vi "DataSender.vi"() -> ()   [LabVIEW 2015]
uses:
  <vilib>/userdefined/High Color/IMAQdx.ctl
  <vilib>/DAQmx/read.llb/DAQmx Read (Analog 2D DBL NChan NSamp).vi
  <vilib>/DAQmx/configure/timing.llb/DAQmx Timing (Sample Clock).vi
  <vilib>/DAQmx/miscellaneous.llb/DAQmx Fill In Error Info.vi
  <vilib>/vision/driver/NI_Vision_Acquisition_Software.lvlib
panel:
  in  "Tab Control 2":T1(tab)
  out "Video Data Acquisition Loop":T2(plugin-control)
  out "Video Display Loop":T2(plugin-control)
  out "Video Save Loop":T2(plugin-control)
  out "AI DAQ Loop":dbl[][](graph)
  out "AI UDP Send & AI Save Loop":dbl[][](graph)
  out ".tdms-file path":path
  out ".bin-file path":path
  out ".avi-file path":path
  in  "Save Binary file":bool
  in  "Save AVI file":bool
  in  "Record Button":bool
  in  "Recording number":dbl
  in  "File path":path
  in  "Stop Button":bool
  in  "Camera module":T3
  # "File paths"
  # "1. Select camera module\n2. Select file path and recording number\n3. Select what file-types to save\n4. Start program\n5. Select \"Record\""
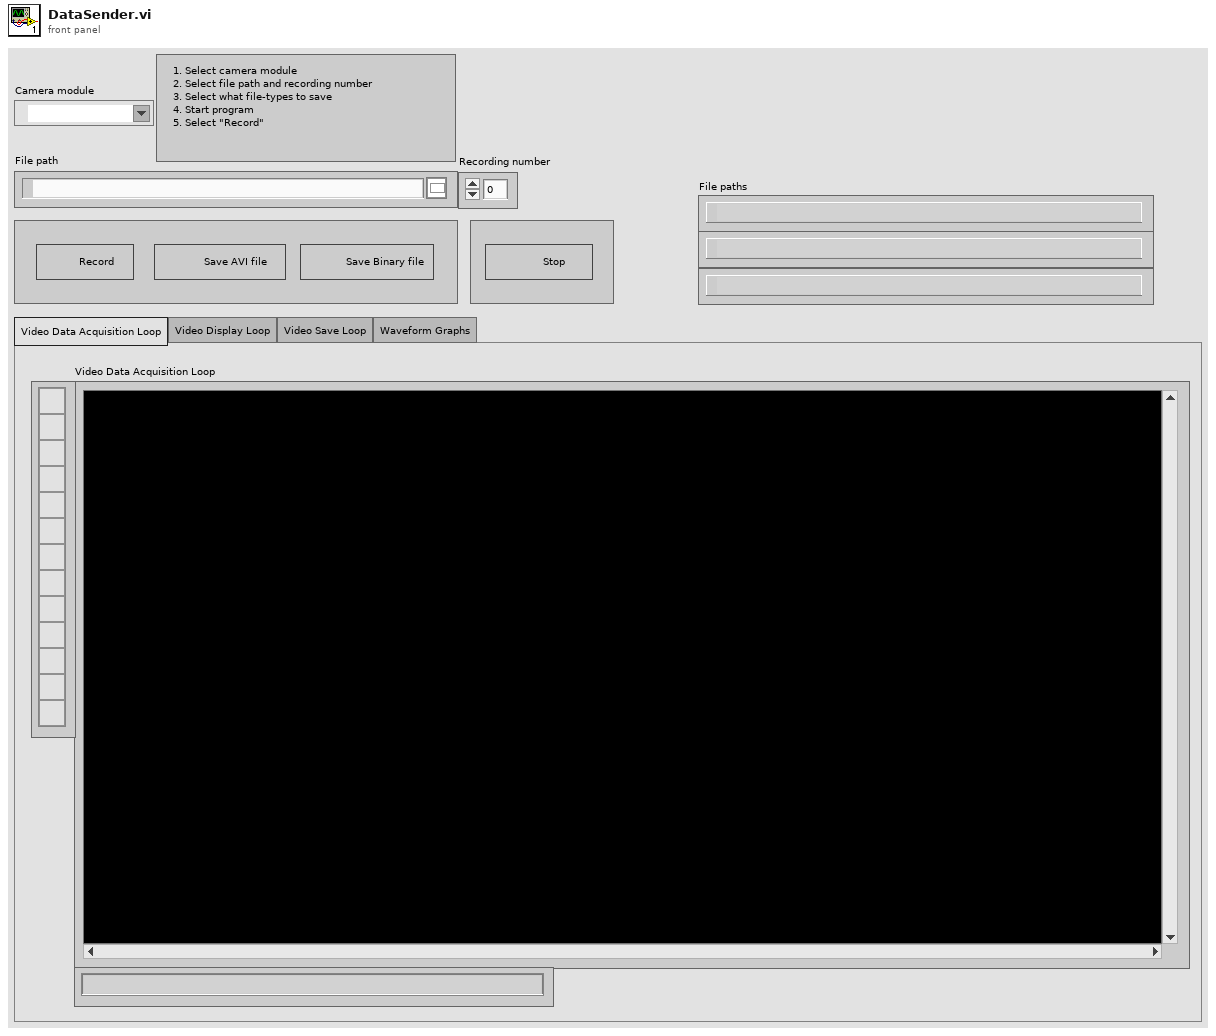
[diagram p1: front panel]
types:
  T1 = enum32{"Video Data Acquisition Loop", "Video Display Loop", "Video Save Loop", "Waveform Graphs"}
  T2 = typedef "IMAQ Image.ctl" = refnum<image>
  T3 = typedef "IMAQdx.ctl" = refnum<k21>
  T4 = enum16{"open", "open or create", "create or replace", "create", "open (read-only)"}
  T5 = enum16{"open", "replace", "create", "open or create", "replace or create", "replace or create with confirmation"}
  T6 = typedef "Image Type" = u32
  T7 = typedef "IMAQ AVI2 Refnum.ctl" = refnum<k20>
  T8 = enum16{"big-endian, network order", "native, host order", "little-endian"}
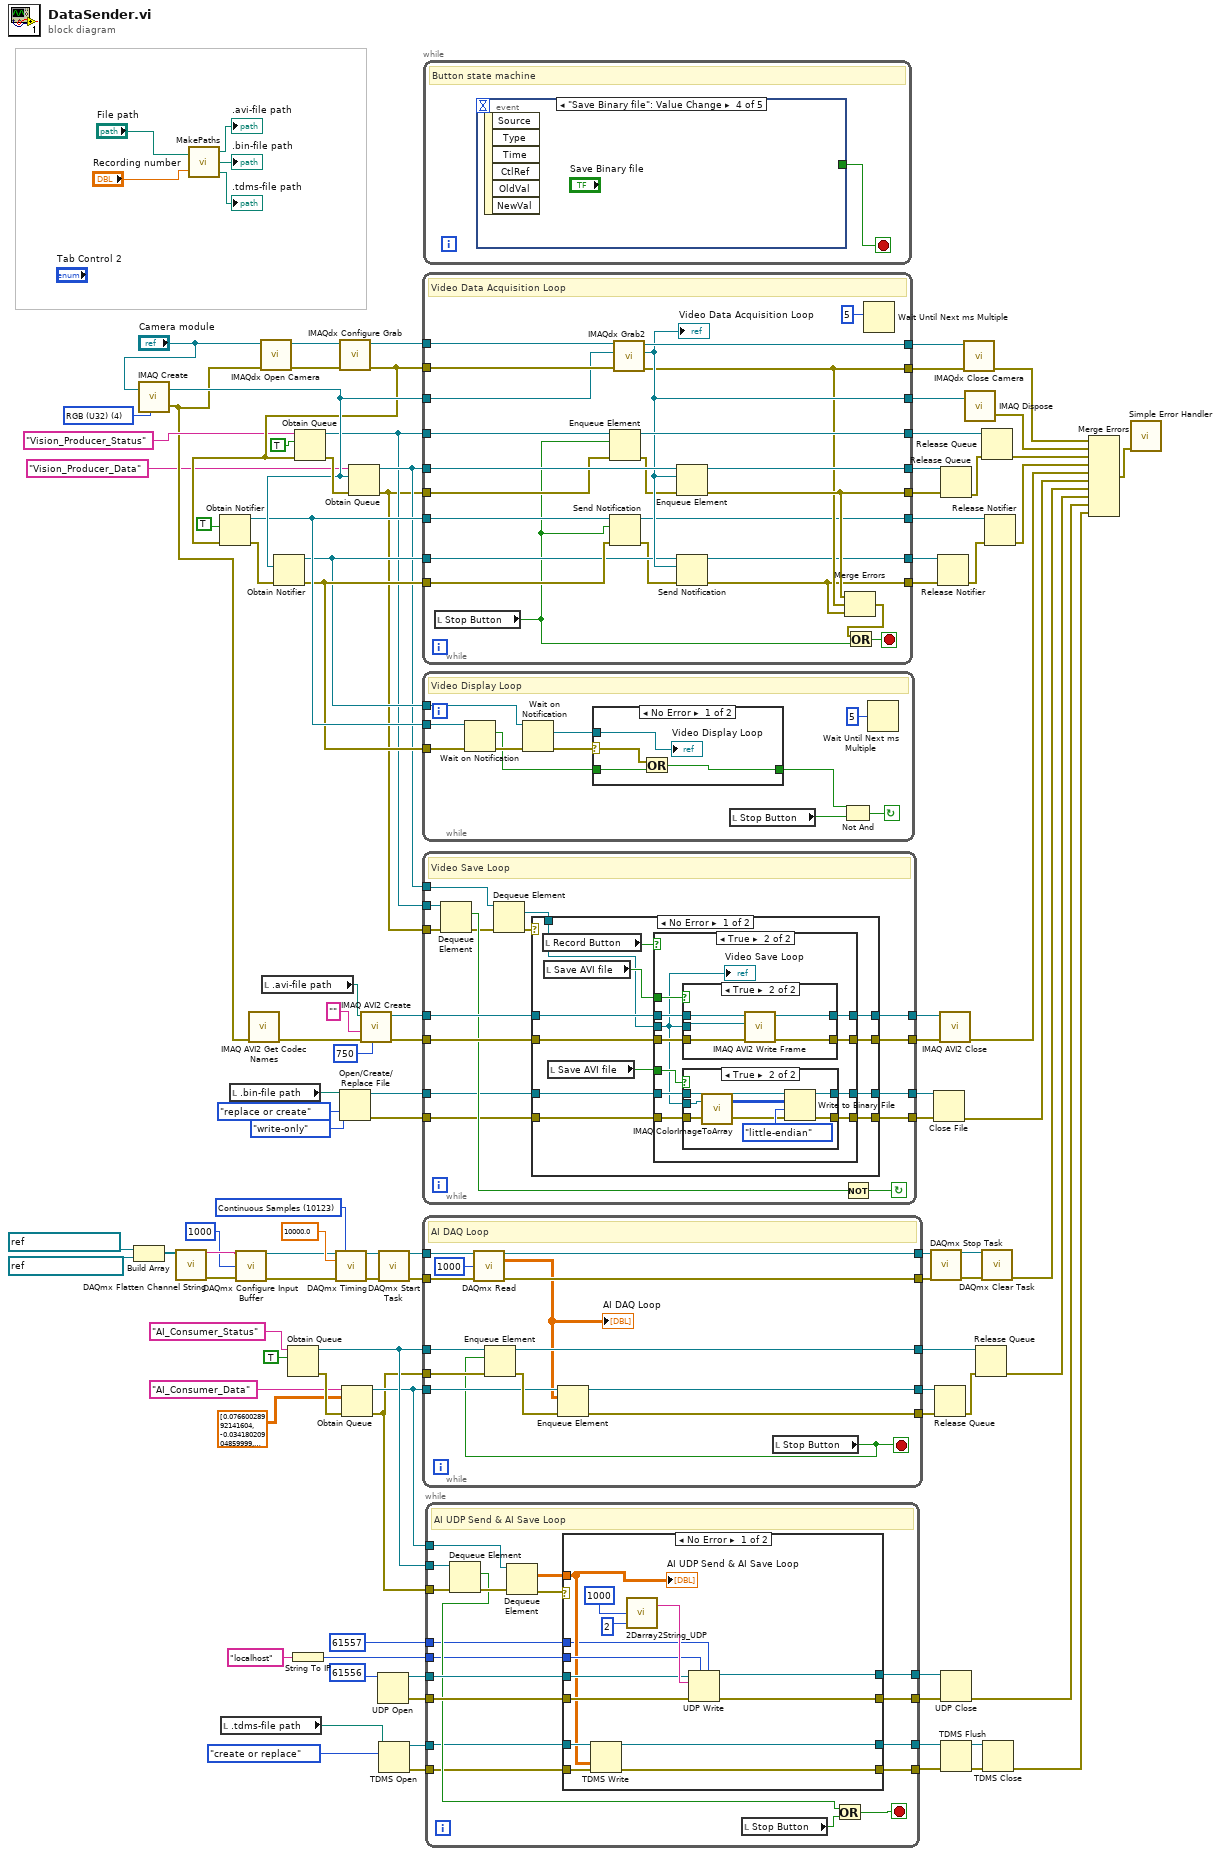
[diagram p0: block diagram]
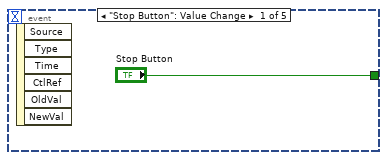
[diagram p2: hidden frame]
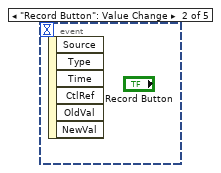
[diagram p3: hidden frame]
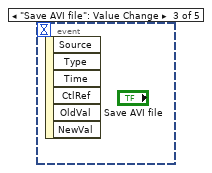
[diagram p4: hidden frame]
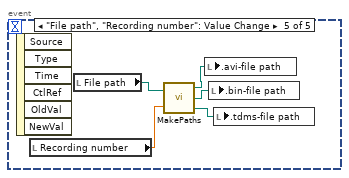
[diagram p5: hidden frame]
diagram:
  w52 = 10123 items=["Finite Samples"=10178, "Continuous Samples"=10123, "Hardware Timed Single Point"=12522] ("sample mode")
  w107 = T6 4 items=["Grayscale (U8)", "Grayscale (I16)", "Grayscale (SGL)", "Complex (CSG)", "RGB (U32)", "HSL (U32)", "RGB (U64)", "Grayscale (U16)"] ("Image Type")
  n1 = Build Array(refnum<k21> "DAQmx_USB_a0" ("global virtual channels"), refnum<k21> "DAQmx_USB_ai1" ("global virtual channels")) -> (w22:refnum<k21>[])
  n2 = call "IMAQ Create"("Image Name"="Camera module", "Image Type"=w107) -> ("New Image"=w85:T2, "error out"=w37:errorcluster)  [unwired: 3 in]
  n3 = call <vilib>:"DAQmx Flatten Channel String.vi"("names in"=w22) -> ("names out"=w21:string, "error out"=w23:errorcluster)  [unwired: 13 in]
  n4 = call "MakePaths.vi"("File path"="File path", "File name index"="Recording number") -> (".avi-file path"=→".avi-file path":path, ".bin-file path"=→".bin-file path":path, ".tdms-file path"=→".tdms-file path":path)
  n5 = local read ".tdms-file path"() -> (w11:path)
  n6 = local read ".bin-file path"() -> (w62:path)
  n7 = call <vilib>:"DAQmx Configure Input Buffer.vi"("task/channels in"=w21, "buffer size (in samples per channel)"=u32 1000, "error in"=w23) -> ("task out"=w25:refnum<k21>, "error out"=w26:errorcluster)  [unwired: 11 in]
  n8 = call "IMAQ AVI2 Get Codec Names"("error in (no error)"=w37) -> ("error out"=w71:errorcluster)  [unwired: 9 in, 1 out]
  n9 = call <vilib>:"IMAQdx Open Camera.vi"("error in"=w37, "Session In"="Camera module") -> ("error out"=w92:errorcluster, "Session Out"=w108:T3)  [unwired: 8 in]
  n10 = local read ".avi-file path"() -> (w68:path)
  n11 = Obtain Queue(name (unnamed)="AI_Consumer_Status", element data type=TRUE) -> (queue out=w29:refnum<queue>, error out=w45:errorcluster)  [unwired: 3 in, 1 out]
  n12 = String To IP(1:"localhost" ("name")) -> (0:w12:u32)
  n13 = call-poly <vilib>:"DAQmx Timing.vi"("task/channels in"=w25, "sample mode"=w52, "rate"=10000.0, "error in"=w26) -> ("task out"=w49:refnum<k21>, "error out"=w48:errorcluster)  [unwired: 10 in]
  n14 = call <vilib>:"IMAQdx Configure Grab.vi"("error in"=w92, "Session In"=w108) -> ("error out"=w76:errorcluster, "Session Out"=w106:T3)  [unwired: 8 in]
  n15 = Obtain Notifier(notification data type=TRUE, error in (no error)=w76) -> (notifier out=w83:refnum<notifier>, error out=w89:errorcluster)  [unwired: 2 in, 1 out]
  n16 = Obtain Notifier(notification data type=w85, error in (no error)=w89) -> (notifier out=w81:refnum<notifier>, error out=w82:errorcluster)  [unwired: 2 in, 1 out]
  n17 = Obtain Queue(name (unnamed)="Vision_Producer_Status", element data type=TRUE, error in (no error)=w76) -> (queue out=w78:refnum<queue>, error out=w101:errorcluster)  [unwired: 2 in, 1 out]
  n18 = Open/Create/Replace File(file path (use dialog)=w62, operation (0:open)=T5."replace or create", access (0:read/write)=enum16{"read/write", "read-only", "write-only"}."write-only") -> (refnum out=w59:refnum<file>, error out=w58:errorcluster)  [unwired: 3 in, 1 out]
  n19 = Obtain Queue(name (unnamed)="AI_Consumer_Data", element data type=dbl[][] [[0.07660028992141604, -0.03418020904859999, 0.11871519035629816, 0.020752269779507133, 0.03143358510719463, 0.10772869459067674, 0.0997940032043946, 0.28046082246128023, 0.10498207064927138, 0.38056000610360874, 0.18097199969481956, 0.30823224231326773, 0.311284046692607, 0.3820859082932784, 0.3564507515068284, 0.4528877698939498, 0.5416952773327229, 0.47669184405279624, 0.6939803158617532, 0.6073090714885175, 0.5560387579156176, 0.5215533684290837, 0.6710917830167086, 0.8279545281147478, 0.7623407339589532, 0.8804455634393835, 0.7989623865110247, 0.942397192339971, 0.7824826428625925, 0.9246967269398032, 0.831616693369955, 0.9442282749675746, 0.9085221637293049, 1.0220492866407263, 1.164568551155871, 0.9750514991989013, 1.0428015564202335, 1.1123826962691692, 1.1206225680933852, 1.1956969558251316, 1.3278400854505226, 1.2719920653086136, 1.3226520180056458, 1.2417792019531548, 1.4630350194552528, 1.2643625543602655, 1.453879606317235, 1.3699549858854048, 1.4087129015030138, 1.4785992217898833, 1.5063706416418707, 1.3907072556649118, 1.6791027695124743, 1.6565194171053637, 1.7166399633783473, 1.58632791638056, 1.7196917677576868, 1.6055542839703976, 1.7880521858548868, 1.7206073090714886, 1.7761501487754634, 1.799649042496376, 1.8023956664377814, 1.731898985275044, 1.9461356527046616, 2.069428549629969, 1.816433966582742, 2.017242694743267, 2.0242618448157472, 1.9760433356221867, 1.9491874570840009, 2.1002517738612956, 2.128023193713283, 2.277256427862974, 2.053864347295338, 2.1911955443656064, 2.317235065232319, 2.3770504310673686, 2.178377965972381, 2.2287327382314794, 2.396887159533074, 2.464637216754406, 2.3141832608529795, 2.3154039826047152, 2.5094987411306935, 2.540627145799954, 2.630655374990463, 2.4350347142748148, 2.4145876249332416, 2.5314717326619363, 2.699931334401465, 2.6623941405355915, 2.75394827191577, 2.589456015869383, 2.705119401846342, 2.656290531776913, 2.6089875638971542, 2.681620508125429, 2.7405203326466774, 2.8427557793545435, 2.938887617303731, 2.9669642175936524, 2.895551995117113, 2.7850766765850308, 3.0130464637216754, 2.8589303425650416, 2.928816662851911, 3.040817883573663, 3.0261692225528343, 2.976729991607538, 3.0283054856183718, 3.0075532158388647, 3.002059967956054, 3.0850690470740827, 3.2593270771343557, 3.1540398260471503, 3.087815671015488, 3.2187380788891433, 3.2001220721751737, 3.241626611734188, 3.4302281223773554, 3.1973754482337684, 3.265430685893034, 3.4296177615014876, 3.3450827801937897, 3.526970321202411, 3.5153734645609216, 3.4726482032501718, 3.36919203479057, 3.4863813229571985, 3.556267643244068, 3.6014343480582895, 3.603875791561761, 3.6066224155031663, 3.5236133363851376, 3.493400473029679, 3.744258793011368, 3.5324635690852215, 3.7558556496528572, 3.8290989547570002, 3.594720378423743, 3.6734569314106964, 3.756466010528725, 3.838864728770886, 3.774166475928893, 3.744258793011368, 3.7390707255664912, 3.833981841763943, 3.9075303273060196, 3.88891432059205, 3.966124971389334, 4.026245517662318, 4.005798428320745, 3.8962386511024643, 3.969787136644541, 4.137026016632334, 3.931334401464866, 4.099183642328526, 4.063172350652323, 4.090638590066376, 3.953612573434043, 4.0650034332799265, 4.038147554741741, 3.9975585564965286, 4.2905317769131, 4.171206225680934, 4.151674677653163, 4.323491264209964, 4.237125200274662, 4.368352788586251, 4.19806210421912, 4.1486228732738235, 4.183108262760357, 4.332341496910048, 4.269779507133593, 4.409857328145266, 4.216983291371023, 4.40161745632105, 4.5053788052185855, 4.436102845807584, 4.417486839093614, 4.305790798809796, 4.425116350041963, 4.365606164644846, 4.4336614023041125, 4.476081483176928, 4.554512855725948, 4.455634393835355, 4.4507515068284125, 4.549324788281071, 4.633249408712902, 4.575570305943389, 4.545052262149996, 4.455329213397421, 4.415960936903945, 4.490424963759823, 4.525520714122225, 4.4925612268253605, 4.654612039368277, 4.630197604333563, 4.563057907988098, 4.6936751354238195, 4.674448767833982, 4.648203250171664, 4.507515068284123, 4.674143587396048, 4.6323338673991, 4.5642786297398334, 4.591744869153887, 4.573434042877851, 4.666208896009766, 4.598764019226367, 4.823376821545739, 4.679026474402991, 4.830090791180285, 4.592355230029755, 4.864576180666819, 4.64240482185092, 4.616464484626535, 4.812390325780117, 4.698252841992828, 4.677500572213321, 4.768139162279698, 4.8490119783321886, 4.8825818265049215, 4.85145342183566, 4.77607385366598, 4.796520943007553, 4.892957961394675, 4.85999847409781, 4.763561455710689, 4.82429236285954, 4.950942244602121, 4.891432059205005, 4.860608834973678, 4.933241779201953, 4.741283283741512, 4.877393759060045, 4.764476997024491, 4.901503013656825, 4.71625848783093, 4.831921873807889, 4.986953536278325, 4.716868848706798, 4.887769893949798, 4.776989394979782, 4.990310521095598, 4.89570458533608, 4.705882352941177, 4.856946669718471, 4.81025406271458, 4.891737239642939, 4.925917448691539, 4.739757381551843, 4.767223620965896, 4.990005340657664, 4.863050278477149, 4.704661631189441, 4.762645914396887, 4.789806973373007, 4.934157320515755, 4.819409475852598, 4.966811627374685, 4.874036774242771, 4.8865491721980625, 4.903028915846495, 4.89021133745327, 4.767223620965896, 4.914930952925918, 4.677805752651255, 4.7440299076829175, 4.680552376592661, 4.866407263294422, 4.70771343556878, 4.889906157015336, 4.743114366369116, 4.831006332494087, 4.8239871824216065, 4.873121232928969, 4.723582818341344, 4.722056916151675, 4.840161745632105, 4.747997253376059, 4.836194399938964, 4.643015182726788, 4.85145342183566, 4.7864499885557334, 4.635996032654307, 4.841077286945906, 4.824902723735408, 4.777294575417716, 4.802014190890364, 4.648508430609598, 4.67505912870985, 4.711070420386053, 4.606393530174715, 4.614023041123064, 4.52674143587396, 4.753795681696803, 4.671702143892577, 4.617380025940337, 4.568551155870908, 4.506904707408255, 4.516975661860075, 4.574959945067521, 4.4885938811322195, 4.5557335774776835, 4.4885938811322195, 4.430914778362707, 4.603341725795376, 4.604562447547112, 4.581368734264133, 4.336308842603189, 4.468757152666514, 4.499885557335775, 4.345464255741207, 4.417486839093614, 4.384222171358816, 4.541390096894789, 4.481574731059739, 4.428473334859236, 4.378423743038072, 4.479438467994202, 4.422674906538491, 4.192874036774243, 4.288090333409628, 4.200503547722591, 4.305180437933928, 4.235294117647059, 4.319218738078889, 4.301213092240787, 4.125429159990845, 4.195315480277714, 4.300907911802853, 4.147402151522088, 4.284733348592355, 4.133363851377127, 4.021057450217441, 4.023498893720912, 4.221560997940032, 4.223086900129702, 4.055237659266041, 4.167849240863661, 3.9319447623407338, 4.028992141603723, 4.078736552986953, 3.9942015716792554, 3.8776226443884947, 4.074158846417944, 4.0683604180972, 3.9047837033646142, 3.8791485465781643, 3.9948119325551232, 3.8907454032196536, 3.986572060730907, 3.6990920881971467, 3.8815899900816357, 3.678644998855573, 3.7973601892118714, 3.812924391546502, 3.7085526817730985, 3.7949187457084, 3.838559548332952, 3.6649118791485464, 3.551384756237125, 3.7839322499427785, 3.616388189517052, 3.714656290531777, 3.689631494621195, 3.60845349813077, 3.489127946898604, 3.467460135805295, 3.4009308003356984, 3.578545815213245, 3.403067063401236, 3.296253910124361, 3.5373464560921644, 3.262989242389563, 3.3157854581521327, 3.4476234073395897, 3.295338368810559, 3.291676203555352, 3.2065308613717862, 3.2382696269169147, 3.167467765316243, 3.143358510719463, 3.2733653772793163, 3.135118638895247, 3.2858777752346073, 3.023117418173495, 3.1204699778744183, 3.1274891279468986, 3.150682841229877, 2.92484931715877, 2.929732204165713, 3.083237964446479, 3.0472266727702753, 2.783245593957427, 3.0218966964217593, 2.994430457007706, 2.9498741130693524, 2.8110170138094146, 2.704509040970474, 2.808575570305943, 2.8140688181887543, 2.827801937895781, 2.6074616617074846, 2.750286106660563, 2.7563897154192416, 2.6706340123598076, 2.7063401235980775, 2.626688029297322, 2.520180056458381, 2.4972915236133364, 2.631876096742199, 2.52475776302739, 2.3300526436255438, 2.374914168001831, 2.469825284199283, 2.491187914854658, 2.434424353398947, 2.354467078660258, 2.2446021210040437, 2.404211490043488, 2.23422598611429, 2.136263065537499, 2.193636987869078, 2.030060273136492, 1.999542229343099, 2.120393682764935, 2.0276188296330204, 2.1680018310826275, 2.0743114366369118, 1.944914930952926, 1.8780804150453956, 1.7834744792858779, 1.9684138246738383, 1.9128709849698635, 1.9336232547493706, 1.9269092851148242, 1.735866330968185, 1.906157015335317, 1.6623178454261083, 1.7419699397268635, 1.7428854810406653, 1.684901197833219, 1.6226443884946975, 1.560387579156176, 1.4209201190203709, 1.3785000381475547, 1.5616083009079118, 1.3830777447165636, 1.509727626459144, 1.5597772182803082, 1.3995574883649957, 1.3528648813611048, 1.385824368657969, 1.4108491645685513, 1.2048523689631494, 1.2091248950942244, 1.0797283894102387, 1.2713817044327458, 1.0522621499961853, 1.134050507362478, 1.0794232089723048, 1.1801327534905013, 1.0730144197756923, 0.9848172732127871, 0.8236820019836728, 0.7989623865110247, 0.788891432059205, 0.9137102311741817, 0.9799343862058442, 0.7284657053482871, 0.7354848554207676, 0.6747539482719158, 0.8114747844663157, 0.7071030746929122, 0.6744487678339819, 0.6198214694438087, 0.5325398641947051, 0.7013046463721675, 0.6884870679789425, 0.48035400930800337, 0.5484092469672694, 0.3811703669794766, 0.36957351033798735, 0.43732356755931945, 0.2865644312199588, 0.28412298771648736, 0.29114213778896775, 0.27862973983367667, 0.21240558480201419, 0.16601815823605706, 0.06805523765926604, 0.24414435034714274, 0.13366903181506065, 0.2404821850919356, 0.2050812542915999, -0.04180971999694819, 0.09308003356984818, -0.09643701838712139, -0.06713969634546425, -0.05035477225909819, -0.05462729839017319, -0.05035477225909819, -0.2697795071335927, -0.24170290684367132, -0.27252613107499807, -0.13031204699778745, -0.16510261692225528, -0.4687571526665141, -0.39032578011749447, -0.45685511558709085, -0.4574654764629587, -0.5957122148470283, -0.5606164644846265, -0.3884946974898909, -0.6094453345540551, -0.6271457999542229, -0.63080796520943, -0.6561379415579461, -0.6671244373235675, -0.652475776302739, -0.8255130846112764, -0.8139162279697871, -0.8014038300144961, -0.8984512092774853, -0.74189364461738, -0.9982452124818799, -0.9579613946746014, -0.9988555733577478, -0.8593881132219425, -1.1035324635690853, -0.9225604638742657, -1.1737239642938888, -1.1590753032730603, -0.9674219882505531, -1.0986495765621425, -1.1221484702830549, -1.0571450370031281, -1.2698558022430761, -1.2961013199053941, -1.4267185473411155, -1.2512397955291066, -1.244831006332494, -1.433127336537728, -1.4721904325932709, -1.4773785000381476, -1.603723201342794, -1.4508278019378957, -1.6742198825055314, -1.6827649347676814, -1.5716792553597314, -1.6403448538948653, -1.6235599298084993, -1.8063630121309224, -1.7364766918440528, -1.582055390249485, -1.6394293125810635, -1.676356145571069, -1.910734721904326, -1.8982223239490348, -1.7389181353475243, -1.9183642328526742, -1.803616388189517, -1.9162279697871367, -1.915312428473335, -1.975127794308385, -2.1097123674372473, -1.9461356527046616, -2.2317845426108187, -2.14023041123064, -2.1054398413061723, -2.0706492713817046, -2.1255817502098115, -2.1045242999923706, -2.1631189440756846, -2.246738384069581, -2.226901655603876, -2.312962539101244, -2.4713511863889526, -2.5189593347066452, -2.38803692683299, -2.4365606164644844, -2.4753185320820936, -2.448767833981842, -2.5256733043411916, -2.6544594491493094, -2.5214007782101167, -2.4512092774853134, -2.67704280155642, -2.6504921034561684, -2.622415503166247, -2.849774929427024, -2.866254673075456, -2.8213931486991686, -2.828717479209583, -2.738078889143206, -2.7856870374608986, -2.8964675364309147, -2.815899900816358, -2.8586251621271077, -2.787518120088502, -3.0722514686808577, -3.0826276035706113, -2.891889829861906, -2.8891432059205004, -3.1573968108644235, -2.9633020523384452, -3.057602807660029, -3.0908674753948273, -3.030746929121843, -3.2504768444342718, -3.130235751888304, -3.2059205004959184, -3.212329289692531, -3.23247119859617, -3.365224689097429, -3.403067063401236, -3.446402685587854, -3.240711070420386, -3.438467994201572, -3.361257343404288, -3.49736781872282, -3.4125276569771876, -3.598687724116884, -3.3380636301213094, -3.4579995422293432, -3.4647135118638897, -3.5315480277714197, -3.5489433127336536, -3.570000762951095, -3.4784466315709164, -3.736324101625086, -3.6606393530174715, -3.5568780041199357, -3.600213626306554, -3.7164873731593806, -3.595025558861677, -3.8702983138780804, -3.851377126726177, -3.880064087891966, -3.8480201419089037, -3.747920958266575, -3.753109025711452, -3.9554436560616466, -3.8190280003051806, -3.884031433585107, -3.8620584420538644, -3.917906462195773, -3.8529030289158466, -3.812924391546502, -4.1199359121080334, -4.128480964370184, -4.096742198825055, -3.9047837033646142, -4.113832303349355, -4.086671244373235, -4.065613794155794, -4.173342488746472, -4.050965133134966, -3.9948119325551232, -4.123292896925307, -4.097047379262989, -4.0442511635004195, -4.334477759975585, -4.075989929045548, -4.352178225375753, -4.111696040283817, -4.356450751506828, -4.275577935454337, -4.158083466849775, -4.287785152971694, -4.282597085526818, -4.437628747997254, -4.436102845807584, -4.246890974288548, -4.320134279392691, -4.373235675593194, -4.480354009308003, -4.539253833829251, -4.389105058365759, -4.529182879377432, -4.440070191500725, -4.341191729610132, -4.560616464484626, -4.54383154039826, -4.615548943312733, -4.415045395590143, -4.4101625085832, -4.616159304188601, -4.566720073243305, -4.483405813687343, -4.581368734264133, -4.583199816891737, -4.43427176317998, -4.615854123750667, -4.563363088426032, -4.615243762874799, -4.571908140688182, -4.627450980392157, -4.779736018921187, -4.518501564049744, -4.691538872358282, -4.789806973373007, -4.590218966964217, -4.655222400244145, -4.624093995574883, -4.556038757915617, -4.606393530174715, -4.571297779812314, -4.587472343022812, -4.695201037613489, -4.617990386816205, -4.740672922865644, -4.670481422140841, -4.742809185931182, -4.631113145647364, -4.819409475852598, -4.729381246662089, -4.761425192645151, -4.822461280231937, -4.713511863889525, -4.695811398489357, -4.814526588845655, -4.7022201876859695, -4.859082932784008, -4.696421759365225, -4.85297932402533, -4.791027695124742, -4.8157473105973905, -4.687571526665141, -4.713817044327459, -4.810864423590448, -4.969558251316091, -4.80018310826276, -4.831311512932021, -4.984817273212787, -4.7525749599450675, -4.897535667963684, -4.961623559929809, -4.753490501258869, -4.872205691615167, -4.847486076142519, -4.817883573662928, -4.900587472343023, -4.854200045777065, -4.903944457160296, -4.8200198367284655, -4.993362325474937, -4.896620126649882, -4.703746089875639, -4.855725947966735, -4.834058136873426, -4.838330663004501, -4.774242771038376, -4.9539940489814605, -4.82429236285954, -4.739757381551843, -4.854505226214999, -4.872510872053101, -4.942092011902037, -4.973525597009232, -4.728160524910353, -4.694895857175555, -4.7318226901655605, -4.931105516136416, -4.868848706797894, -4.943617914091707, -4.905470359349966, -4.840161745632105, -4.799267566948958, -4.7022201876859695, -4.857251850156405, -4.6939803158617535, -4.860914015411612, -4.653086137178607, -4.790722514686808, -4.794384679942016, -4.798046845197223, -4.82581826504921, -4.658274204623484, -4.607614251926451, -4.85297932402533, -4.8578622110322724, -4.712901503013657, -4.730296787975891, -4.574349584191653, -4.669565880827039, -4.673228046082246, -4.770885786221103, -4.737926298924239, -4.6494239719234, -4.799267566948958, -4.641794460975052, -4.579842832074464, -4.753185320820935, -4.682688639658198, -4.764171816586557, -4.542000457770657, -4.615548943312733, -4.549324788281071, -4.585641260395208, -4.630197604333563, -4.673838406958114, -4.5725185015640495, -4.510872053101396, -4.38605325398642, -4.4043640802624555, -4.599984740978103, -4.6436255436026554, -4.46845197222858, -4.57099259937438, -4.594796673533226, -4.542000457770657, -4.450141145952545, -4.486152437628748, -4.285954070344091, -4.285954070344091, -4.325932707713435, -4.486152437628748, -4.433051041428245, -4.457160296025025, -4.333867399099717, -4.315556572823682, -4.303349355306325, -4.432135500114443, -4.286869611657893, -4.327458609903105, -4.361943999389639, -4.086976424811169, -4.220340276188296, -4.09399557488365, -4.272220950637064, -4.114747844663157, -4.249027237354086, -4.130922407873656, -4.011596856641489, -4.056458381017777, -4.238345922026398, -4.133058670939193, -4.198367284657054, -4.042114900434882, -3.8873884184023804, -4.023804074158846, -4.130006866559854, -3.9472037842374306, -3.8245212481879913, -3.9163805600061035, -3.8367284657053484, -3.859616998550393, -3.8159761959258414, -3.8867780575265125, -3.8443579766536966, -3.7595178149080644, -3.786068513008316, -3.8614480811779965, -3.8525978484779126, -3.613031204699779, -3.7506675822079805, -3.615777828641184, -3.624322880903334, -3.5754940108339057, -3.5629816128786147, -3.7839322499427785, -3.6862745098039214, -3.71099412527657, -3.671625848783093, -3.6853589684901196, -3.4448767833981844, -3.5205615320057984, -3.59136339360647, -3.458304722667277, -3.312428473334859, -3.3868925001907377, -3.4857709620813306, -3.3112077515831233, -3.347829404135195, -3.42748149843595, -3.4644083314259557, -3.1815060654612037, -3.2062256809338523, -3.3627832455939575, -3.2895399404898145, -3.1119249256122683, -3.105516136415656, -3.096971084153506, -3.096971084153506, -3.134813458457313, -3.1024643320363166, -3.1100938429846647, -3.0304417486839093, -2.972457465476463, -3.0823224231326773, -2.862287327382315, -2.98619058518349, -3.0469214923323413, -2.860761425192645, -2.9132524605172807, -2.771343556878004, -2.9053177691309986, -2.6977950713359276, -2.6501869230182344, -2.6746013580529486, -2.75547417410544, -2.725871671625849, -2.631876096742199, -2.6507972838941023, -2.7148851758602275, -2.4884412909132525, -2.5433737697413594, -2.5137712672617685, -2.4713511863889526, -2.392004272526131, -2.563210498207065, -2.5473411154345005, -2.558022430762188, -2.2708476386663614, -2.444190127412833, -2.4243533989471273, -2.4386968795300223, -2.1640344853894864, -2.205233844510567, -2.341039139391165, -2.3074692912184327, -2.3044174868390934, -2.0364690623331043, -2.161287861448081, -1.999542229343099, -2.020904859998474, -2.0178530556191348, -1.876249332417792, -2.115205615320058, -2.0526436255436025, -1.9476615548943312, -1.8744182497901885, -1.9555962462806133, -1.8771648737315938, -1.8863202868696116, -1.8243686579690241, -1.7727931639581902, -1.6473640039673456, -1.6116578927290761, -1.7715724422064545, -1.530174715800717, -1.5463492790112154, -1.684596017395285, -1.5454337376974137, -1.5762569619287403, -1.5497062638284886, -1.3311970702677958, -1.4813458457312887, -1.3315022507057297, -1.3034256504158084, -1.2353704127565424, -1.4520485236896314, -1.3864347295338368, -1.313191424429694, -1.3415732051575493, -1.215228503852903, -1.2143129625391011, -1.2463569085221637, -1.1749446860456245, -1.1703669794766156, -1.1932555123216602, -1.0464637216754407, -0.8703746089875639, -0.8300907911802854, -0.8438239108873121, -0.959792477302205, -0.814526588845655, -0.7034409094377051, -0.7772945754177157, -0.7754634927901122, -0.8026245517662318, -0.6912336919203479, -0.5569542992294194, -0.6765850308995194, -0.5035477225909819, -0.6942854962996872, -0.5722133211261158, -0.4058899824521248, -0.6420996414129855, -0.4342717631799802, -0.42481116960402837, -0.341191729610132, -0.3909361409933623, -0.2868696116578927, -0.42786297398336764, -0.2859540703440909, -0.2743572137026017, -0.12756542305638208, -0.21637293049515527, -0.17120622568093385, -0.08819714656290532, -0.08941786831464103, -0.1718165865568017, 0.0311284046692607, 0.07171740291447318], [0.35065232318608375, 0.5310139620050355, 0.42481116960402837, 0.4852368963149462, 0.6454566262302587, 0.5859464408331426, 0.6515602349889372, 0.614023041123064, 0.5719081406881819, 0.8090333409628443, 0.5972381170366979, 0.7992675669489586, 0.7244983596551461, 0.9539940489814603, 0.7129015030136568, 0.8853284504463264, 0.7559319447623407, 1.0629434653238727, 1.1139085984588388, 1.0727092393377584, 0.899977111467155, 1.0861371786068512, 1.1740291447318227, 1.2591744869153887, 1.134050507362478, 1.142900740062562, 1.2561226825360494, 1.3156328679331655, 1.279011215381094, 1.2173647669184404, 1.1795223926146334, 1.4032196536202028, 1.4358739604791333, 1.4917219806210422, 1.4267185473411155, 1.4251926451514458, 1.560997940032044, 1.5188830395971618, 1.6870374608987564, 1.7169451438162813, 1.6778820477607386, 1.530174715800717, 1.5368886854352637, 1.6739147020675975, 1.8261997405966277, 1.6830701152056153, 1.7578393224994278, 1.718165865568017, 1.7502098115510796, 1.944914930952926, 1.7935454337376975, 1.9983215075913634, 1.8222323949034867, 2.013275349050126, 2.041962310215915, 2.032806897077897, 2.205233844510567, 2.1768520637827113, 1.9867246509498742, 2.1850919356069274, 2.0520332646677346, 2.1100175478751813, 2.2662699320973525, 2.1805142290379185, 2.3434805828946366, 2.408178835736629, 2.2781719691767757, 2.358434424353399, 2.461585412375067, 2.558327611200122, 2.3236438544289313, 2.5626001373311973, 2.502784771496147, 2.549477378500038, 2.4875257495994507, 2.5690089265278098, 2.626993209735256, 2.716716258487831, 2.7576104371709773, 2.5503929198138398, 2.7444876783398184, 2.7277027542534524, 2.8799877927824826, 2.6800946059357593, 2.8418402380407417, 2.7023727779049365, 2.8522163729304952, 2.771648737315938, 3.0417334248874646, 2.87357900358587, 2.8546578164339667, 2.8561837186236363, 3.105210955977722, 2.981307698176547, 2.9187457084000914, 3.19829098954757, 3.1665522240024413, 3.2089723048752576, 3.231860837720302, 3.1488517586022735, 3.3093766689555197, 3.3533226520180057, 3.282520790417334, 3.3344014648661022, 3.1778439002059966, 3.2346074616617075, 3.4396887159533076, 3.385976958876936, 3.426871137560082, 3.441519798580911, 3.2718394750896467, 3.303578240634775, 3.308155947203784, 3.4171053635461965, 3.5025558861676966, 3.658808270389868, 3.3969634546425573, 3.4787518120088503, 3.5040817883573663, 3.735713740749218, 3.551995117112993, 3.577630273899443, 3.6279850461585412, 3.608148317692836, 3.615777828641184, 3.595025558861677, 3.6737621118486303, 3.855344472419318, 3.8522926680399787, 3.6774242771038375, 3.794613565270466, 3.813839932860304, 3.9209582665751124, 4.005798428320745, 3.940489814602884, 3.768978408484016, 3.9890135042343786, 4.007324330510414, 3.9395742732890824, 3.881284809643702, 4.080872816052491, 3.999084458686198, 3.9157701991302356, 4.052796215762569, 4.065918974593728, 4.1739528496223395, 4.145571068894484, 4.128786144808118, 3.982299534599832, 4.221866178377966, 4.050659952697032, 4.138857099259938, 4.0988784618905925, 4.1879911497673, 4.22919050888838, 4.2746623941405355, 4.116273746852826, 4.169985503929198, 4.323796444647898, 4.30457007705806, 4.202029449912261, 4.351567864499885, 4.227664606698711, 4.226443884946975, 4.267338063630121, 4.473640039673457, 4.428168154421302, 4.3585870145723655, 4.476691844052796, 4.544441901274128, 4.586861982146944, 4.566720073243305, 4.599984740978103, 4.385137712672618, 4.558785381857023, 4.429388876173038, 4.5975432974746315, 4.414129854276341, 4.548104066529335, 4.641184100099184, 4.646677347981995, 4.667734798199436, 4.700999465934234, 4.552071412222476, 4.6018158236057065, 4.460517280842298, 4.736705577172503, 4.545967803463798, 4.695201037613489, 4.780956740672923, 4.516670481422141, 4.5557335774776835, 4.77454795147631, 4.725719081406882, 4.648813611047532, 4.715648126955062, 4.776379034103914, 4.570382238498512, 4.732433051041428, 4.852063782711528, 4.638437476157779, 4.679636835278859, 4.638742656595713, 4.6103608758678565, 4.850537880521858, 4.753490501258869, 4.627756160830091, 4.821545738918135, 4.639658197909514, 4.909742885481041, 4.906691081101702, 4.703440909437705, 4.696421759365225, 4.70771343556878, 4.921034561684596, 4.802014190890364, 4.836194399938964, 4.906080720225834, 4.7864499885557334, 4.86854352635996, 4.698252841992828, 4.758678568703746, 4.957656214236668, 4.775158312352178, 4.78461890592813, 4.75043869687953, 4.733043411917296, 4.867322804608224, 4.8325322346837565, 4.866407263294422, 4.698863202868696, 4.854810406652933, 4.9286640726329445, 4.703135728999771, 4.709544518196384, 4.838025482566567, 4.856641489280537, 4.813305867093919, 4.906691081101702, 4.8743419546807045, 4.985732814526589, 4.790722514686808, 4.9747463187609675, 4.880445563439384, 4.794995040817883, 4.69214923323415, 4.934157320515755, 4.873426413366903, 4.7348744945449, 4.694285496299687, 4.771496147096971, 4.946669718471046, 4.827954528114748, 4.792858777752346, 4.710154879072252, 4.686655985351339, 4.804455634393835, 4.834973678187228, 4.913099870298314, 4.725413900968948, 4.8783093003738465, 4.890516517891204, 4.928969253070878, 4.730296787975891, 4.75898374914168, 4.762951094834821, 4.671396963454643, 4.732127870603494, 4.799877927824826, 4.73334859235523, 4.837415121690699, 4.690318150606546, 4.787060349431601, 4.845349813076981, 4.664072632944229, 4.694895857175555, 4.563057907988098, 4.827954528114748, 4.821240558480201, 4.608529793240253, 4.689097428854811, 4.652475776302739, 4.642710002288854, 4.64240482185092, 4.744640268558785, 4.530098420691234, 4.49408712901503, 4.472114137483787, 4.664682993820096, 4.645761806668193, 4.579232471198596, 4.491340505073625, 4.61371786068513, 4.629587243457695, 4.3833066300450145, 4.4000915541313805, 4.599374380102235, 4.565804531929503, 4.55390249485008, 4.534065766384375, 4.419928282597086, 4.539253833829251, 4.319523918516823, 4.5297932402533, 4.553292133974212, 4.519111924925612, 4.343938353551537, 4.426642252231632, 4.380254825665675, 4.281071183337148, 4.221866178377966, 4.307011520561532, 4.347905699244678, 4.265812161440452, 4.208743419546807, 4.274967574578469, 4.267643244068055, 4.375371938658732, 4.288090333409628, 4.170901045243, 4.053711757076371, 4.307927061875334, 4.179140917067216, 4.22369726100557, 4.197146562905318, 4.227359426260777, 3.979247730220493, 3.9423208972304877, 4.1779201953154805, 3.975280384527352, 3.944762340733959, 4.042420080872816, 3.9145494773785, 4.114442664225223, 4.009460593575952, 3.9118028534370946, 4.051575494010834, 4.014953841458762, 3.940794995040818, 3.913939116502632, 3.8834210727092393, 3.8739604791332876, 3.8321507591363395, 3.8272678721293967, 3.817502098115511, 3.776913099870298, 3.735408560311284, 3.722590981918059, 3.6725413900968946, 3.6911573968108646, 3.6279850461585412, 3.680170901045243, 3.7174029144731824, 3.5025558861676966, 3.718623636224918, 3.539787899595636, 3.6435492484931715, 3.385671778439002, 3.591973754482338, 3.5938048371099414, 3.3792629892423895, 3.312428473334859, 3.488212405584802, 3.51293202105745, 3.3383688105592433, 3.2001220721751737, 3.2220950637064165, 3.4119172961013198, 3.2062256809338523, 3.39330128938735, 3.2382696269169147, 3.1525139238574806, 3.1662470435645074, 3.0869001297016863, 3.005416952773327, 3.1836423285267412, 3.061264972915236, 2.98466468299382, 3.0463111314564735, 3.019455252918288, 3.092698558022431, 2.895857175555047, 2.8061341268024718, 3.0536354619668877, 2.7579156176089112, 2.968490119783322, 2.7600518806744487, 2.8131532768749525, 2.8253604943923096, 2.861982146944381, 2.6535439078355076, 2.8479438467994203, 2.845502403295949, 2.754863813229572, 2.7862973983367665, 2.758525978484779, 2.601968413824674, 2.592813000686656, 2.6285191119249256, 2.561684596017395, 2.3974975204089417, 2.5705348287174794, 2.477759975585565, 2.293125810635538, 2.478675516899367, 2.4554818036163883, 2.452124818799115, 2.247348744945449, 2.1988250553139546, 2.145113298237583, 2.120393682764935, 2.0556954299229417, 2.2168307011520563, 2.264744029907683, 2.272068360418097, 2.20157167925536, 1.9339284351873045, 2.1002517738612956, 1.9214160372320135, 1.9729915312428474, 2.069733730067903, 2.0706492713817046, 1.9513237201495384, 1.952849622339208, 1.8731975280384527, 1.736171511406119, 1.8954757000076294, 1.7468528267338064, 1.7721828030823223, 1.7453269245441367, 1.5545891508354315, 1.6488899061570153, 1.5613031204699779, 1.6189822232394904, 1.454184786755169, 1.6427862973983367, 1.6260013733119707, 1.471274891279469, 1.5365835049973298, 1.3443198290989549, 1.5045395590142672, 1.369039444571603, 1.3925383382925154, 1.176775768673228, 1.1883726253147173, 1.3281452658884565, 1.1288624399176013, 1.1883726253147173, 1.258258945601587, 1.0473792629892424, 1.0754558632791638, 1.1029221026932174, 0.959487296864271, 0.8801403830014496, 0.9274433508812086, 1.0116731517509727, 0.8142214084077211, 0.7437247272449836, 0.7269398031586175, 0.9002822919050889, 0.7696650644693676, 0.8651865415426871, 0.6811627374685283, 0.814526588845655, 0.7879758907454032, 0.7650873579003585, 0.7174792095826658, 0.4620431830319677, 0.5673304341191729, 0.3799496452277409, 0.3781185626001373, 0.354009308003357, 0.5069047074082551, 0.3204394598306249, 0.24963759822995346, 0.281376363775082, 0.3054856183718624, 0.3689631494621195, 0.1330586709391928, 0.2316319523918517, 0.2975509269855802, 0.11169604028381781, 0.24811169604028382, 0.13977264057373923, 0.13031204699778745, -0.08789196612497138, 0.07690547035934997, -0.019836728465705347, -0.12695506218051422, -0.1815823605706874, -0.05493247882810712, -0.10620279240100709, -0.03143358510719463, -0.2887006942854963, -0.35919737544823377, -0.24719615472648204, -0.2801556420233463, -0.21332112611581597, -0.2307164110780499, -0.33600366216525523, -0.2859540703440909, -0.4217593652246891, -0.4528877698939498, -0.3915465018692302, -0.5136186770428015, -0.5838101777676051, -0.5676356145571069, -0.5795376516365301, -0.5828946364538033, -0.7769893949797818, -0.7058823529411765, -0.8987563897154193, -0.929579613946746, -0.8520637827115282, -0.9826810101472495, -0.8276493476768139, -0.8310063324940872, -0.9607080186160067, -0.8538948653391317, -1.0333409628442818, -0.8941786831464104, -1.1480888075074387, -1.1349660486762798, -1.1459525444419012, -1.0070954451819638, -1.2054627298390173, -1.1819638361181048, -1.091020065613794, -1.249713893339437, -1.3864347295338368, -1.437094682230869, -1.4874494544899672, -1.270771343556878, -1.2848096437018388, -1.4343480582894637, -1.6092164492256047, -1.4261081864652476, -1.376974135957885, -1.6690318150606547, -1.5042343785763332, -1.4767681391622798, -1.5243762874799724, -1.5286488136110474, -1.6821545738918136, -1.6549935149156938, -1.8393224994277866, -1.68886854352636, -1.8600747692072939, -1.8869306477454795, -2.0148012512397955, -1.9681086442359044, -2.0721751735713743, -1.8817425803006027, -2.1136797131303884, -2.1475547417410543, -1.9430838483253223, -2.08194094758526, -2.124361028458076, -2.153047989623865, -2.021820401312276, -2.1768520637827113, -2.0746166170748457, -2.1991302357518885, -2.379186694132906, -2.276035706111238, -2.4118410009918363, -2.2949568932631417, -2.367284657053483, -2.2497901884489204, -2.5424582284275576, -2.3147936217288474, -2.4426642252231634, -2.527504386968795, -2.6376745250629434, -2.6279087510490577, -2.6498817425803005, -2.461280231937133, -2.6968795300221258, -2.5943389028763257, -2.5702296482795455, -2.5516136415655755, -2.7780575265125504, -2.6205844205386435, -2.72983901731899, -2.7350270847638667, -2.8882276646066987, -2.8796826123445487, -2.973067826352331, -3.0337987335011825, -2.836652170595865, -2.890974288548104, -2.8973830777447165, -2.9706263828488595, -2.951400015259022, -3.1665522240024413, -3.1494621194781414, -3.0420386053253985, -3.257190814068818, -3.216601815823606, -3.0862897688258184, -3.1570916304264895, -3.2169069962615398, -3.117723353933013, -3.1964599069199666, -3.138170443274586, -3.2352178225375754, -3.2474250400549325, -3.2858777752346073, -3.483329518577859, -3.424429694056611, -3.3746852826733806, -3.3237201495384148, -3.3920805676356145, -3.5324635690852215, -3.5196459906919966, -3.653620202944991, -3.5526054779888607, -3.4351110093842983, -3.570611123826963, -3.6652170595864804, -3.493095292591745, -3.587701228351263, -3.7671473258564125, -3.72808422980087, -3.693598840314336, -3.6432440680552376, -3.6429388876173037, -3.790951400015259, -3.7625696192874036, -3.7296101319905395, -3.9337758449683373, -3.740291447318227, -3.8736552986953536, -3.8904402227817196, -3.945372701609827, -4.021972991531243, -4.067139696345464, -3.7894254978255892, -3.9862668802929733, -3.8275730525673306, -4.1113908598458835, -3.876096742198825, -4.1611352712291145, -4.040283817807278, -3.93011367971313, -4.113832303349355, -4.027771419851987, -4.14526588845655, -3.9884031433585108, -4.171511406118868, -4.015259021896696, -4.202029449912261, -4.144960708018616, -4.176699473563745, -4.107728694590676, -4.3793392843518735, -4.263065537499046, -4.231631952391852, -4.286259250782025, -4.151064316777295, -4.187075608453498, -4.192263675898375, -4.336919203479057, -4.458686198214695, -4.281071183337148, -4.3082322423132675, -4.519417105363546, -4.430609597924773, -4.4272526131075, -4.327153429465171, -4.398870832379645, -4.368657969024185, -4.490424963759823, -4.360723277637903, -4.339665827420462, -4.495002670328832, -4.44281681544213, -4.513008316166934, -4.56244754711223, -4.561837186236362, -4.451667048142214, -4.471198596169986, -4.46295872434577, -4.623788815136949, -4.6308079652094305, -4.559395742732891, -4.594186312657358, -4.5725185015640495, -4.7519645990692, -4.654306858930343, -4.710154879072252, -4.533455405508507, -4.52124818799115, -4.565194171053635, -4.771801327534905, -4.627145799954223, -4.716563668268864, -4.672312504768445, -4.7177843900206, -4.6897077897306785, -4.688181887541009, -4.732433051041428, -4.7946898603799495, -4.858777752346074, -4.621957732509346, -4.744640268558785, -4.652170595864805, -4.620126649881742, -4.763561455710689, -4.8783093003738465, -4.7986572060730905, -4.817883573662928, -4.907911802853437, -4.763866636148623, -4.721141374837873, -4.826733806363012, -4.7486076142519265, -4.847180895704585, -4.866712443732356, -4.7864499885557334, -4.790722514686808, -4.705271992065309, -4.686350804913405, -4.7989623865110245, -4.827038986800946, -4.924086366063936, -4.842603189135576, -4.988784618905928, -4.77454795147631, -4.740672922865644, -4.876783398184177, -4.924696726939803, -4.876783398184177, -4.745860990310521, -4.742504005493248, -4.805371175707637, -4.964980544747082, -4.75043869687953, -4.799572747386892, -4.805065995269703, -4.884107728694591, -4.914625772487984, -4.868848706797894, -4.984817273212787, -4.880750743877318, -4.737315938048371, -4.754100862134737, -4.864576180666819, -4.753795681696803, -4.7107652399481195, -4.721446555275807, -4.7568474860761425, -4.766918440527962, -4.936293583581293, -4.7440299076829175, -4.964980544747082, -4.723887998779278, -4.903639276722362, -4.909742885481041, -4.943312733653773, -4.806897077897307, -4.730296787975891, -4.889295796139468, -4.817883573662928, -4.876783398184177, -4.8661020828564885, -4.867627985046158, -4.772716868848707, -4.635690852216373, -4.859388113221942, -4.6390478370336465, -4.696421759365225, -4.652170595864805, -4.785534447241932, -4.762951094834821, -4.691844052796216, -4.650339513237202, -4.8368047608148315, -4.684214541847868, -4.648203250171664, -4.759288929579614, -4.577096208133058, -4.712596322575723, -4.6771953917753875, -4.625619897764554, -4.557869840543221, -4.669565880827039, -4.607919432364385, -4.589913786526283, -4.596017395284962, -4.592660410467689, -4.649118791485466, -4.423895628290227, -4.415350576028077, -4.506599526970321, -4.5093461509117265, -4.430609597924773, -4.549935149156939, -4.453192950331884, -4.583810177767605, -4.408331425955597, -4.510261692225528, -4.486457618066682, -4.399176012817579, -4.3750667582207985, -4.511787594415198, -4.328984512092775, -4.3253223468375674, -4.356450751506828, -4.465705348287175, -4.191042954146639, -4.247196154726482, -4.436408026245518, -4.432135500114443, -4.352483405813687, -4.298466468299382, -4.170595864805066, -4.137331197070268, -4.1071183337148085, -4.0610360875867855, -4.0607309071488515, -4.250858319981689, -4.267643244068055, -4.121766994735637, -3.9929808499275197, -4.028076600289921, -4.237430380712596, -3.9975585564965286, -4.038452735179675, -4.011596856641489, -4.1400778210116735, -3.918211642633707, -4.015869382772564, -3.8995956359197375, -3.9145494773785, -3.875486381322957, -3.9169909208819713, -3.9722285801480126, -3.871519035629816, -3.830319676508736, -3.995117112993057, -3.7845426108186464, -3.7122148470283056, -3.887998779278248, -3.914244296940566, -3.818417639429313, -3.6108949416342413, -3.83062485694667, -3.662775616083009, -3.799496452277409, -3.7582970931563286, -3.5156786449988555, -3.5294117647058822, -3.675898374914168, -3.5684748607614254, -3.534905012588693, -3.4396887159533076, -3.657587548638132, -3.547722590981918, -3.43755245288777, -3.4573891813534754, -3.322804608224613, -3.526665140764477, -3.51445792324712, -3.347219043259327, -3.3804837109941253, -3.253833829251545, -3.245593957427329, -3.299610894941634, -3.202563515678645, -3.253223468375677, -3.309071488517586, -3.1201647974364843, -3.1113145647364004, -3.2422369726100557, -3.0554665445944913, -3.1778439002059966, -3.03593499656672, -2.9144731822690164, -3.039291981383993, -2.919661249713893, -2.9266803997863735, -2.9825284199282827, -3.0200656137941557, -2.9456015869382774, -2.8342107270923935, -2.886091401541161, -2.9187457084000914, -2.845502403295949, -2.6501869230182344, -2.660563057907988, -2.8418402380407417, -2.601358052948806, -2.7106126497291525, -2.6675822079804683, -2.7661554894331273, -2.7481498435950256, -2.563210498207065, -2.691386282139315, -2.4853894865339132, -2.400854505226215, -2.3941405355916685, -2.4933241779201953, -2.4194705119401845, -2.341344319829099, -2.3196765087357902, -2.332494087129015, -2.288853284504463, -2.3694209201190204, -2.2406347753109026, -2.2458228427557794, -2.1466392004272525, -2.2149996185244527, -2.256504158083467, -2.1942473487449456, -2.178072785534447, -2.11459525444419, -2.1463340199893186, -1.8673990997177081, -1.8588540474555582, -1.8481727321278707, -2.0071717402914473, -1.9543755245288776, -1.778286411841001, -1.8393224994277866, -1.9598687724116883, -1.774013885709926, -1.8234531166552224, -1.8197909514000152, -1.8136873426413367, -1.6696421759365225, -1.7264057373922332, -1.5530632486457618, -1.595178149080644, -1.466086823834592, -1.5747310597390707, -1.5234607461661707, -1.4395361257343404, -1.5881589990081635, -1.3836881055924315, -1.4853131914244297, -1.4438086518654154, -1.4428931105516136, -1.2295719844357977, -1.377279316395819, -1.1822690165560388, -1.0629434653238727, -1.0485999847409782, -1.2973220416571298, -0.9866483558403907, -1.2133974212252994, -0.9961089494163424, -1.1395437552452887, -1.0855268177309834, -1.0623331044480049, -0.8688487067978943, -0.7959105821316853, -1.0080109864957656, -0.9097428854810407, -0.6894026092927443, -0.9182879377431906, -0.7513542381933318, -0.6845197222858015, -0.6540016784924086, -0.6445410849164569, -0.7071030746929122, -0.4992751964599069, -0.4422064545662623, -0.6854352635996033, -0.6536964980544747, -0.5697718776226444, -0.588387884336614, -0.37628747997253376, -0.5099565117875944, -0.49713893339436943, -0.2178988326848249, -0.38879987792782483, -0.15014877546349278, -0.31158922713054094, -0.14312962539101243, -0.30731670099946595, -0.08331425955596246, 0.021057450217441064, -0.22339208056763563, -0.06530861371786069, 0.0057984283207446405, -0.07019150072480354, 0.011596856641489281, 0.15259021896696423, 0.05371175707637141, 0.007019150072480354, 0.17883573662928207, 0.04852368963149462, 0.2511635004196231, 0.21454184786755168, 0.29327840085450524, 0.285648889906157, 0.2166781109330892, 0.2264438849469749, 0.25879301136797134]] ("Waveform Graph 3"), error in (no error)=w45) -> (queue out=w28:refnum<queue>, error out=w27:errorcluster)  [unwired: 2 in, 1 out]
  n20 = Obtain Queue(name (unnamed)="Vision_Producer_Data", element data type=w85, error in (no error)=w101) -> (queue out=w79:refnum<queue>, error out=w77:errorcluster)  [unwired: 2 in, 1 out]
  n21 = call "IMAQ AVI2 Create"("Quality"=750, "error in (no error)"=w71, "Codec"="", "AVI Path"=w68) -> ("error out"=w74:errorcluster, "AVI Refnum"=w75:T7)  [unwired: 6 in]
  n22 = UDP Open(11:u16 61556 ("port")) -> (port=w13:refnum<k16>, 0:w16:errorcluster)  [unwired: 4 in, 1 out]
  n23 = call <vilib>:"DAQmx Start Task.vi"("task/channels in"=w49, "error in"=w48) -> ("task out"=w24:refnum<k21>, "error out"=w47:errorcluster)  [unwired: 12 in]
  n24 = TDMS Open(10:T4."create or replace" ("operation (0:open)"), 11:w11) -> (0:w8:errorcluster, 3:w9:refnum<k34>)  [unwired: 5 in]
  n25 = while {
    tunnel: w106 -> [w132]
    tunnel: w76 -> [w131]
    tunnel: w85 -> [w130]
    tunnel: [w129] -> w104
    tunnel: [w120] -> w105
    tunnel: [w123] -> w103
    tunnel: w78 -> [w128]
    tunnel: [w127] -> w100
    tunnel: w79 -> [w126]
    tunnel: w77 -> [w125]
    tunnel: [w124] -> w99
    tunnel: [w121] -> w98
    tunnel: w83 -> [w117]
    tunnel: [w116] -> w91
    tunnel: w82 -> [w115]
    tunnel: [w114] -> w88
    tunnel: w81 -> [w113]
    tunnel: [w112] -> w84
    stop <- w118 stop-if-true
    # "Video Data Acquisition Loop"
    n26 = local read "Stop Button"() -> (w111:bool)
    n27 = Enqueue Element(queue=w128, element=w111, error in (no error)=w125) -> (queue out=w127:refnum<queue>, error out=w110:errorcluster)  [unwired: 1 in, 1 out]
    n28 = Send Notification(notification=w111, notifier=w117, error in (no error)=w115) -> (notifier out=w116:refnum<notifier>, error out=w109:errorcluster)
    n29 = call <vilib>:"IMAQdx Grab2.vi"("error in"=w131, "Image In"=w130, "Session In"=w132) -> ("error out"=w120:errorcluster, "Image Out"=w123:T2, "Session Out"=w129:T3)  [unwired: 5 in, 1 out]
    "Video Data Acquisition Loop" <- w123
    n30 = Enqueue Element(queue=w126, element=w123, error in (no error)=w110) -> (queue out=w124:refnum<queue>, error out=w121:errorcluster)  [unwired: 1 in, 1 out]
    n31 = Send Notification(notification=w123, notifier=w113, error in (no error)=w109) -> (notifier out=w112:refnum<notifier>, error out=w114:errorcluster)
    n32 = Merge Errors(w121, w120, w114) -> (w119:errorcluster)
    n33 = Or(x=w119, y=w111) -> (x .or. y?=w118:bool)
    n34 = Wait Until Next ms Multiple(millisecond multiple=u32 5) -> ()  [unwired: 1 out]
  }
  n35 = while {
    tunnel: w83 -> [w142]
    tunnel: w82 -> [w141]
    tunnel: w81 -> [w140]
    stop <- w139 continue-if-true
    # "Video Display Loop"
    n36 = Wait on Notification(notifier=w142, error in (no error)=w141) -> (notification=w136:bool, error out=w143:errorcluster)  [unwired: 2 in, 2 out]
    n37 = Wait on Notification(notifier=w140, error in (no error)=w143) -> (notification=w137:T2, error out=w138:errorcluster)  [unwired: 2 in, 2 out]
    n38 = case shown="No Error" w138 {
      selector: w138 -> [w146 _]
      tunnel: w137 -> [w147 _]
      tunnel: w136 -> [w145 w148]
      tunnel: [w144 w148] -> w133
      frame No Error {
        n39 = Or(x=w146, y=w145) -> (x .or. y?=w144:bool)
        "Video Display Loop" <- w147
      }
      frame Error {
      }
    }
    n40 = local read "Stop Button"() -> (w135:bool)
    n41 = Not And(1:w133, 2:w135) -> (0:w139:bool)
    n42 = Wait Until Next ms Multiple(millisecond multiple=u32 5) -> ()  [unwired: 1 out]
  }
  n43 = while {
    tunnel: w79 -> [w164]
    tunnel: w78 -> [w163]
    tunnel: w77 -> [w162]
    tunnel: w75 -> [w161]
    tunnel: w74 -> [w160]
    tunnel: [w159] -> w73
    tunnel: [w158] -> w72
    tunnel: w59 -> [w152]
    tunnel: w58 -> [w151]
    tunnel: [w150] -> w57
    tunnel: [w149] -> w56
    stop <- w157 continue-if-true
    # "Video Save Loop"
    n44 = Dequeue Element(queue=w163, error in (no error)=w162) -> (element=w156:bool, error out=w155:errorcluster)  [unwired: 1 in, 2 out]
    n45 = Dequeue Element(queue=w164, error in (no error)=w155) -> (element=w154:T2, error out=w153:errorcluster)  [unwired: 1 in, 2 out]
    n46 = case shown="No Error" w153 {
      tunnel: w161 -> [w176 w212]
      tunnel: w160 -> [w175 w211]
      tunnel: [w174 w211] -> w159
      tunnel: [w173 w212] -> w158
      tunnel: w154 -> [w171 _]
      tunnel: w152 -> [w168 w210]
      tunnel: w151 -> [w167 w209]
      tunnel: [w166 w210] -> w150
      tunnel: [w165 w209] -> w149
      frame No Error {
        n47 = local read "Record Button"() -> (w170:bool)
        n48 = local read "Save AVI file"() -> (w172:bool)
        n49 = local read "Save AVI file"() -> (w169:bool)
        n50 = case shown="True" w170 {
          tunnel: w176 -> [w180 w191]
          tunnel: w175 -> [w179 w190]
          tunnel: [w179 w189] -> w174
          tunnel: [w180 w188] -> w173
          tunnel: w172 -> [_ w187]
          tunnel: w171 -> [_ w181]
          tunnel: w169 -> [_ w186]
          tunnel: w168 -> [w178 w185]
          tunnel: w167 -> [w177 w184]
          tunnel: [w178 w183] -> w166
          tunnel: [w177 w182] -> w165
          frame False {
          }
          frame True {
            n51 = case shown="True" w187 {
              tunnel: w191 -> [w203 w208]
              tunnel: w190 -> [w202 w207]
              tunnel: [w202 w206] -> w189
              tunnel: [w203 w205] -> w188
              tunnel: w181 -> [_ w204]
              frame False {
              }
              frame True {
                n52 = call "IMAQ AVI2 Write Frame"("error in (no error)"=w207, "Image"=w204, "AVI Refnum"=w208) -> ("error out"=w206:errorcluster, "AVI Refnum (duplicate)"=w205:T7)  [unwired: 6 in, 1 out]
              }
            }
            n53 = case shown="True" w186 {
              tunnel: w185 -> [w193 w201]
              tunnel: w184 -> [w192 w196]
              tunnel: [w193 w200] -> w183
              tunnel: [w192 w199] -> w182
              tunnel: w181 -> [_ w197]
              frame False {
              }
              frame True {
                n54 = call "IMAQ ColorImageToArray"("Image"=w197, "error in (no error)"=w196) -> ("Image Pixels (U32)"=w194:u32[][], "error out"=w195:errorcluster)  [unwired: 2 in, 1 out]
                n55 = Write to Binary File(file (use dialog)=w201, data=w194, error in=w195, 9:T8."little-endian" ("byte order (0:big-endian, network order)")) -> (refnum out=w200:refnum<file>, error out=w199:errorcluster)  [unwired: 2 in, 1 out]
              }
            }
            "Video Save Loop" <- w181
          }
        }
      }
      frame Error {
      }
    }
    n56 = Not(x=w156) -> (.not. x?=w157:bool)
  }
  n57 = while {
    tunnel: [w226] -> w35
    tunnel: [w225] -> w34
    tunnel: w24 -> [w224]
    tunnel: w47 -> [w223]
    tunnel: w29 -> [w222]
    tunnel: [w221] -> w43
    tunnel: w27 -> [w220]
    tunnel: [w218] -> w42
    tunnel: w28 -> [w216]
    tunnel: [w217] -> w41
    stop <- w215 stop-if-true
    # "AI DAQ Loop"
    n58 = call-poly <vilib>:"DAQmx Read.vi"("task/channels in"=w224, "number of samples per channel"=1000, "error in"=w223) -> ("task out"=w225:refnum<k21>, "data"=w213:dbl[][], "error out"=w226:errorcluster)  [unwired: 10 in]
    "AI DAQ Loop" <- w213
    n59 = local read "Stop Button"() -> (w215:bool)
    n60 = Enqueue Element(queue=w222, element=w215, error in (no error)=w220) -> (queue out=w221:refnum<queue>, error out=w219:errorcluster)  [unwired: 1 in, 1 out]
    n61 = Enqueue Element(queue=w216, element=w213, error in (no error)=w219) -> (queue out=w217:refnum<queue>, error out=w218:errorcluster)  [unwired: 1 in, 1 out]
  }
  n62 = while {
    stop <- w227 stop-if-true
    # "Button state machine"
    n63 = event shown="[3] \"Save Binary file\": Value Change" {
      selector: _ -> [_ _ _ _ _]
      dyn-events: _ -> [_ _ _ _ _]
      timeout: _ -> [_ _ _ _ _]
      tunnel: ["Stop Button" _ _ _ _] -> w227
      event "Stop Button": Value Change {
        n64 = event-data() -> ()  [unwired: 1 in, 6 out]
      }
      event "Record Button": Value Change {
        n65 = event-data() -> ()  [unwired: 1 in, 6 out]
      }
      event "Save AVI file": Value Change {
        n66 = event-data() -> ()  [unwired: 1 in, 6 out]
      }
      event "Save Binary file": Value Change {
        n67 = event-data() -> ()  [unwired: 1 in, 6 out]
      }
      event "File path", "Recording number": Value Change {
        n68 = event-data() -> ()  [unwired: 1 in, 6 out]
        n69 = local read "Recording number"() -> (w233:dbl)
        n70 = local read "File path"() -> (w232:path)
        n71 = call "MakePaths.vi"("File path"=w232, "File name index"=w233) -> (".avi-file path"=w231:path, ".bin-file path"=w230:path, ".tdms-file path"=w229:path)
        n72 = local write ".avi-file path"(w231) -> ()
        n73 = local write ".bin-file path"(w230) -> ()
        n74 = local write ".tdms-file path"(w229) -> ()
      }
    }
  }
  n75 = while {
    tunnel: w29 -> [w252]
    tunnel: w28 -> [w251]
    tunnel: w27 -> [w250]
    tunnel: w16 -> [w244]
    tunnel: [w243] -> w15
    tunnel: [w242] -> w14
    tunnel: w13 -> [w241]
    tunnel: w12 -> [w239]
    tunnel: w9 -> [w238]
    tunnel: w8 -> [w237]
    tunnel: [w236] -> w5
    tunnel: [w235] -> w4
    tunnel: u16 61557 ("port or service name") -> [w234]
    stop <- w248 stop-if-true
    # "AI UDP Send & AI Save Loop"
    n76 = Dequeue Element(queue=w252, error in (no error)=w250) -> (element=w240:bool, error out=w249:errorcluster)  [unwired: 1 in, 2 out]
    n77 = Dequeue Element(queue=w251, error in (no error)=w249) -> (element=w245:dbl[][], error out=w246:errorcluster)  [unwired: 1 in, 2 out]
    n78 = case shown="No Error" w246 {
      tunnel: w245 -> [w256 _]
      tunnel: w244 -> [w263 w269]
      tunnel: [w262 w269] -> w243
      tunnel: [w261 w270] -> w242
      tunnel: w241 -> [w260 w270]
      tunnel: w239 -> [w259 _]
      tunnel: w238 -> [w258 w268]
      tunnel: w237 -> [w257 w267]
      tunnel: [w255 w268] -> w236
      tunnel: [w254 w267] -> w235
      tunnel: w234 -> [w253 _]
      frame No Error {
        n79 = TDMS Write(0:w258, 9:w256, 11:w257) -> (4:w255:refnum<k34>, 15:w254:errorcluster)  [unwired: 3 in, 2 out]
        n80 = call "2Darray2String_UDP.vi"("NumberOfChannels"=2, "NumberOfSamples"=1000) -> ("UDP_String"=w264:string)  [unwired: 1 in, 1 out]
        n81 = UDP Write(address=w259, port or service name=w253, connection ID=w260, data in=w264, 8:w263) -> (error out=w262:errorcluster, 3:w261:refnum<k16>)  [unwired: 1 in]
        "AI UDP Send & AI Save Loop" <- w256
      }
      frame Error {
      }
    }
    n82 = local read "Stop Button"() -> (w247:bool)
    n83 = Or(x=w240, y=w247) -> (x .or. y?=w248:bool)
  }
  n84 = call <vilib>:"DAQmx Stop Task.vi"("task/channels in"=w34, "error in"=w35) -> ("task out"=w33:refnum<k21>, "error out"=w32:errorcluster)  [unwired: 12 in]
  n85 = Close File(refnum=w57, error in=w56) -> (error out=w54:errorcluster)  [unwired: 1 out]
  n86 = Release Queue(queue=w41, error in (no error)=w42) -> (error out=w44:errorcluster)  [unwired: 1 in, 2 out]
  n87 = Release Notifier(notifier=w84, error in (no error)=w88) -> (error out=w87:errorcluster)  [unwired: 1 in, 2 out]
  n88 = call "IMAQ AVI2 Close"("error in (no error)"=w73, "AVI Refnum"=w72) -> ("error out"=w55:errorcluster)  [unwired: 9 in]
  n89 = Release Queue(queue=w99, error in (no error)=w98) -> (error out=w97:errorcluster)  [unwired: 1 in, 2 out]
  n90 = UDP Close(connection ID=w14, 8:w15) -> (error out=w3:errorcluster)  [unwired: 1 out]
  n91 = TDMS Flush(4:w4, 7:w5) -> (0:w7:errorcluster, 3:w6:refnum<k34>)
  n92 = call <vilib>:"IMAQdx Close Camera.vi"("error in"=w105, "Session In"=w104) -> ("error out"=w94:errorcluster)  [unwired: 9 in]
  n93 = call "IMAQ Dispose"("Image"=w103) -> ("error out"=w95:errorcluster)  [unwired: 5 in]
  n94 = Release Queue(queue=w43, error in (no error)=w44) -> (error out=w30:errorcluster)  [unwired: 1 in, 2 out]
  n95 = Release Queue(queue=w100, error in (no error)=w97) -> (error out=w93:errorcluster)  [unwired: 1 in, 2 out]
  n96 = call <vilib>:"DAQmx Clear Task.vi"("task in"=w33, "error in"=w32) -> ("error out"=w31:errorcluster)  [unwired: 13 in]
  n97 = TDMS Close(8:w7, 11:w6) -> (0:w2:errorcluster)  [unwired: 1 out]
  n98 = Release Notifier(notifier=w91, error in (no error)=w87) -> (error out=w86:errorcluster)  [unwired: 1 in, 2 out]
  n99 = Merge Errors(w94, w95, w93, w86, w55, w54, w31, w30, w3, w2) -> (w96:errorcluster)
  n100 = call <vilib>:"Simple Error Handler.vi"("error in (no error)"=w96) -> ()  [unwired: 4 in, 5 out]
